vi "CrawlingState.vi"(8 "error in (no error)":errorcluster, 9 "Cluster in":T2, 10 "Enum in":T1, 11 "Actual Start [i]":i64) -> (0 "error out":errorcluster, 2 "Cluster out":T2, 3 "Enum":T1)   [LabVIEW 2018]
uses:
  Type_Def Actuator Controls.ctl
  Type_Def_ControlState.ctl
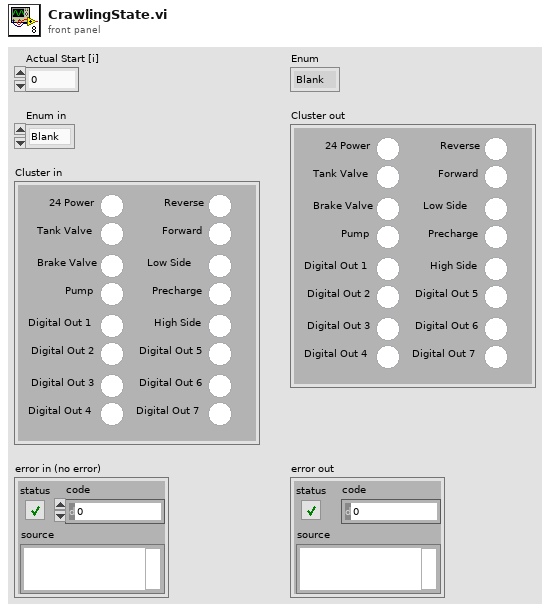
[diagram p1: front panel]
types:
  T1 = typedef "Type_Def_ControlState.ctl" = enum16{"Blank", "Systems Check", "Idle", "Ready", "Pushing", "CrawlingPrecharge", "Braking", "Fault", "Boot Up", "Unpowered", "Crawling", "Shutdown", "Service Push", "Service Wait", "Vent", "Precharge", "Cooldown"}
  T2 = typedef "Type_Def Actuator Controls.ctl" = cluster{"Reverse ":bool, "Forward":bool, "Low Side":bool, "Precharge":bool, "High Side":bool, "Digital Out 5":bool, "Digital Out 6":bool, "Digital Out 7 ":bool, "24 Power":bool, "Tank Valve ":bool, "Brake Valve":bool, "Pump":bool, "Digital Out 1 ":bool, "Digital Out 2":bool, "Digital Out 3":bool, "Digital Out 4 ":bool}
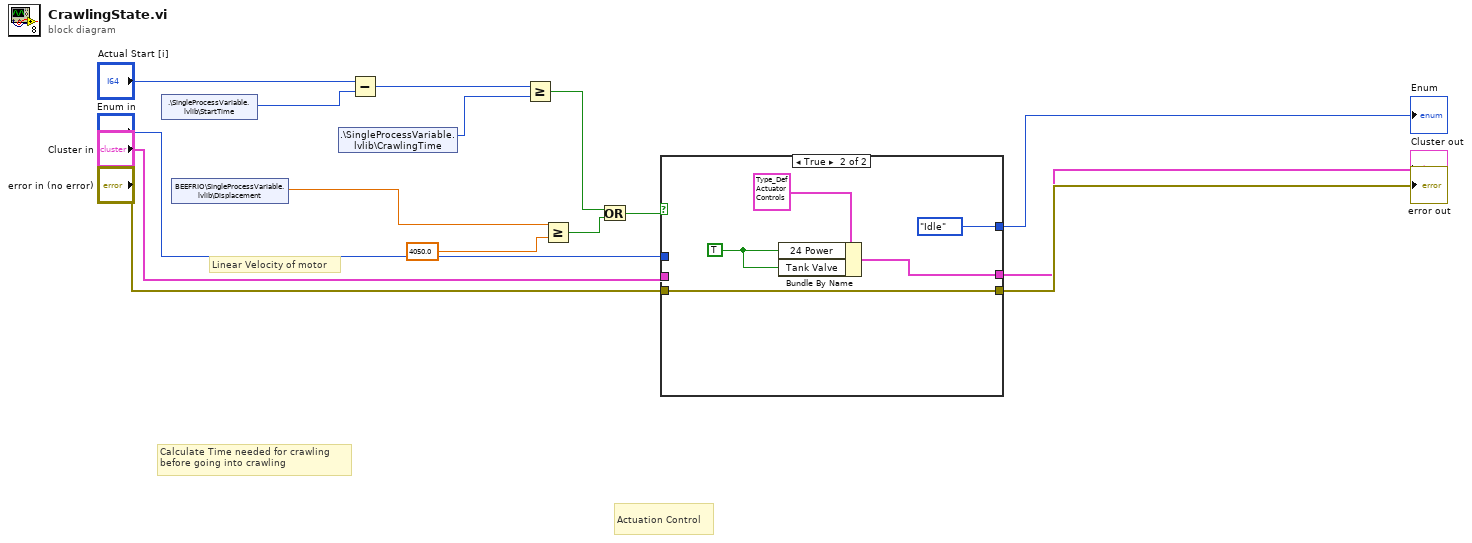
[diagram p0: block diagram]
diagram:
  # "Calculate Time needed for crawling \nbefore going into crawling"
  # "Linear Velocity of motor"
  # "Actuation Control"
  n1 = shared-variable ".\\SingleProcessVariable.lvlib\\StartTime"() -> (w8:i64)  [unwired: 1 in, 1 out]
  n2 = shared-variable "BEEFRIO\\SingleProcessVariable.lvlib\\Displacement"() -> (w14:dbl)  [unwired: 1 in, 1 out]
  n3 = shared-variable ".\\SingleProcessVariable.lvlib\\CrawlingTime"() -> (w15:i64)  [unwired: 1 in, 1 out]
  n4 = Subtract(x="Actual Start [i]", y=w8) -> (x-y=w9:i64)
  n5 = Greater Or Equal?(x=w9, y=w15) -> (x >= y?=w10:bool)
  n6 = Greater Or Equal?(x=w14, y=4050.0) -> (x >= y?=w12:bool)
  n7 = Or(x=w10, y=w12) -> (x .or. y?=w13:bool)
  n8 = case shown="True" w13 {
    tunnel: "Enum in" -> [w18 _]
    tunnel: [w18 Type_Def_ControlState."Idle"] -> w2
    tunnel: "Cluster in" -> [w17 _]
    tunnel: [w17 w22] -> w4
    tunnel: [w16 w21] -> w5
    tunnel: "error in (no error)" -> [w16 w21]
    frame False {
    }
    frame True {
      w20 = TRUE ("Brake Valve")
      n9 = Bundle By Name(cluster=T2 {"Reverse "=FALSE, "Forward"=FALSE, "Low Side"=FALSE, "Precharge"=FALSE, "High Side"=FALSE, "Digital Out 5"=FALSE, "Digital Out 6"=FALSE, "Digital Out 7 "=FALSE, "24 Power"=FALSE, "Tank Valve "=FALSE, "Brake Valve"=FALSE, "Pump"=FALSE, "Digital Out 1 "=FALSE, "Digital Out 2"=FALSE, "Digital Out 3"=FALSE, "Digital Out 4 "=FALSE} ("Cluster in 2"), "24 Power"=w20, "Tank Valve"=w20) -> (w22:T2)
    }
  }
  "error out" <- w5
  "Cluster out" <- w4
  "Enum" <- w2
